vi "标样核查.vi"(11 "标样核查配置":T1={"数据保存间隔"=1.0, "水温标样值"=0.0, "pH标样值"=0.0, "溶解氧标样值"=0.0, "电导率标样值"=0.0, "浊度标样值"=0.0}) -> ()   [LabVIEW 2016, in "国弘多参数.lvlib"]
panel:
  out "运行状态":u16(ring) items=["空闲", "水样测试", "标样核查"]
  out "seconds since 1Jan1904":timestamp
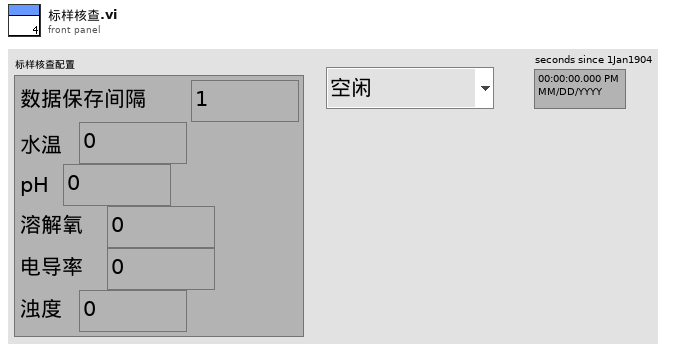
[diagram p1: front panel]
types:
  T1 = cluster{"数据保存间隔":dbl, "水温标样值":dbl, "pH标样值":dbl, "溶解氧标样值":dbl, "电导率标样值":dbl, "浊度标样值":dbl}
  T2 = cluster{"因子编码":string, "单位":string, "标样参考值":sgl, "水样数据时间":timestamp, "水样实测值":sgl, "水样数据标识":string, "探头温度":sgl}
  T3 = typedef "LVDateTimeRec.ctl" = cluster{"秒数的小数部分":dbl, "秒":i32, "分":i32, "时":i32, "日":i32, "月":i32, "年":i32, "天数（周）":i32, "天数（年）":i32, "DST":i32}
  T4 = cluster{"CH":u16, "监测值":dbl, "监测信号值":dbl, "温度偏移修正值":sgl}
  T5 = cluster{"电极状态标志":u16, "电极型号标志":u16, "酸碱度测量值":sgl, "温度测量值":sgl, "酸碱度信号值":sgl, "温度信号值":sgl, "酸碱度偏移修正值":sgl, "温度偏移修正值":sgl, "手动温度补偿值":sgl, "酸碱度电极零点":sgl, "酸碱度电极斜率":sgl, "第1点标准值记录":sgl, "第1点信号值记录":sgl, "第1点温度值记录":sgl, "第2点标准值记录":sgl, "第2点信号值记录":sgl, "第2点温度值记录":sgl, "命令滤波设定":u16, "温度模式":enum16{"ATC", "MTC"}, "生产批次":u16, "电极序号":u16, "串口地址":u16, "串口波特率":enum16{"9600", "19200", "115200"}, "串口校验位":enum16{"NONE", "ODD", "EVEN"}, "串口停止位":enum16{"1bit", "2bit"}, "第一点标准值":sgl, "第二点标准值":sgl}
  T6 = cluster{"电极状态标志":u16, "电极型号标志":u16, "溶解氧测量值":sgl, "温度测量值":sgl, "溶解氧饱和度值":sgl, "盐度补偿值":sgl, "大气压补偿值":sgl, "溶解氧偏移修正值":sgl, "温度偏移修正值":sgl, "手动温度补偿值":sgl, "溶解氧电极零点":sgl, "溶解氧电极斜率":sgl, "第1点标准值记录":sgl, "第1点信号值记录":sgl, "第1点温度值记录":sgl, "第2点标准值记录":sgl, "第2点信号值记录":sgl, "第2点温度值记录":sgl, "命令滤波设定":u16, "温度模式":enum16{"ATC", "MTC"}, "生产批次":u16, "电极序号":u16, "串口地址":u16, "串口波特率":enum16{"9600", "19200", "115200"}, "串口校验位":enum16{"NONE", "ODD", "EVEN"}, "串口停止位":enum16{"1bit", "2bit"}, "第一点标准值":sgl, "第二点标准值":sgl}
  T7 = cluster{"电极状态标志":u16, "电极型号标志":u16, "电导率测量值":sgl, "温度测量值":sgl, "电导率信号值":sgl, "温度信号值":sgl, "温度补偿系数":sgl, "电导率偏移修正值":sgl, "温度偏移修正值":sgl, "手动温度补偿值":sgl, "电导率电极零点":sgl, "电导率电极斜率":sgl, "命令滤波设定":u16, "温度模式":enum16{"ATC", "MTC"}, "生产批次":u16, "电极序号":u16, "串口地址":u16, "串口波特率":enum16{"9600", "19200", "115200"}, "串口校验位":enum16{"NONE", "ODD", "EVEN"}, "串口停止位":enum16{"1bit", "2bit"}, "第一点标准值":sgl, "第二点标准值":sgl}
  T8 = cluster{"电极状态标志":u16, "电极型号标志":u16, "浊度测量值":sgl, "温度测量值":sgl, "浊度信号值":sgl, "浊度偏移修正值":sgl, "温度偏移修正值":sgl, "手动温度补偿值":sgl, "浊度电极零点":sgl, "浊度电极斜率":sgl, "第1点标准值记录":sgl, "第1点信号值记录":sgl, "第1点温度值记录":sgl, "第2点标准值记录":sgl, "第2点信号值记录":sgl, "第2点温度值记录":sgl, "命令滤波设定":u16, "温度模式":enum16{"ATC", "MTC"}, "生产批次":u16, "电极序号":u16, "串口地址":u16, "串口波特率":enum16{"9600", "19200", "115200"}, "串口校验位":enum16{"NONE", "ODD", "EVEN"}, "串口停止位":enum16{"1bit", "2bit"}, "第一点标准值":sgl, "第二点标准值":sgl}
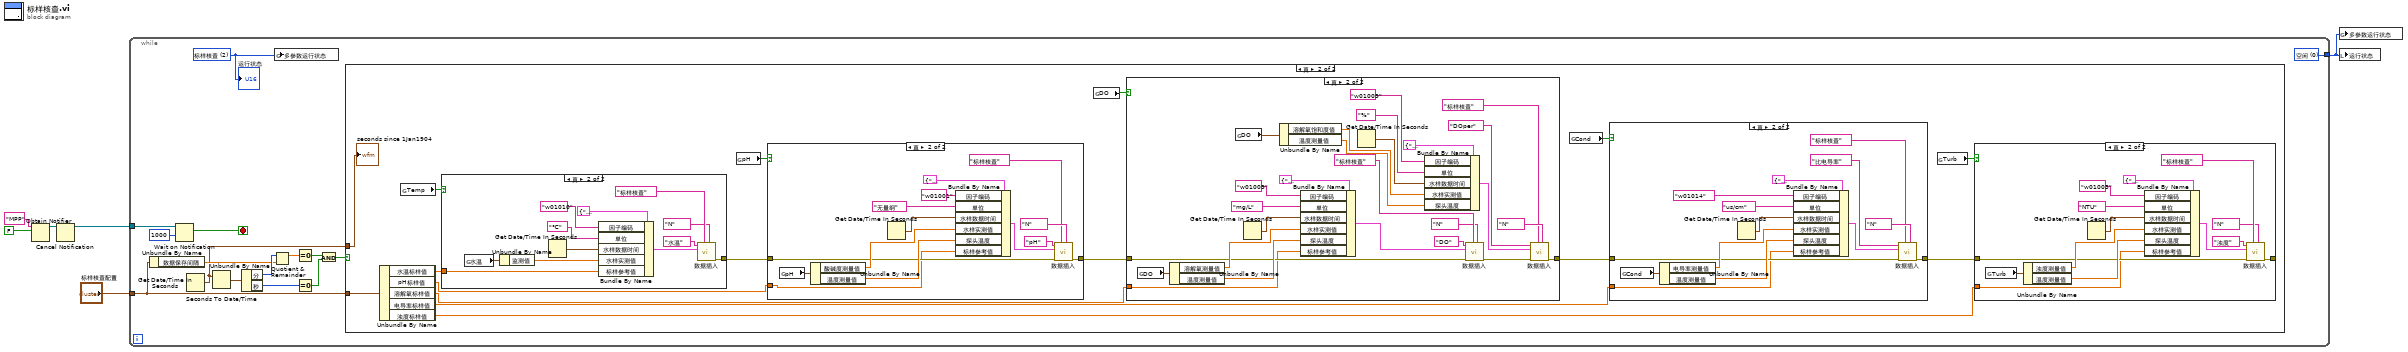
[diagram p0: block diagram]
diagram:
  n1 = Obtain Notifier(name (unnamed)="MPP" ("名称（未命名）"), notification data type=FALSE) -> (notifier out=w2:refnum<notifier>)  [unwired: 2 in, 2 out]
  n2 = Cancel Notification(0:w2) -> (8:w1:refnum<notifier>)  [unwired: 1 in, 2 out]
  n3 = while {
    tunnel: "标样核查配置" -> [w17]
    tunnel: [w11] -> w5
    tunnel: w1 -> [w9]
    stop <- w7 stop-if-true
    w11 = u16 0 items=["空闲", "水样测试", "标样核查"] ("多参数运行状态")
    w10 = u16 2 items=["空闲", "水样测试", "标样核查"] ("多参数运行状态")
    n4 = Unbundle By Name(w17) -> ("数据保存间隔"=w15:dbl)
    n5 = Wait on Notification(notifier=w9, timeout in ms (-1)=1000 ("超时毫秒(-1)")) -> (notification=w7:bool)  [unwired: 2 in, 3 out]
    n6 = Get Date/Time In Seconds() -> (seconds since 1Jan1904=w12:timestamp)
    n7 = Seconds To Date/Time(time stamp (now)=w12) -> (date time rec=w21:T3)  [unwired: 1 in]
    n8 = Unbundle By Name(w21) -> ("分"=w16:i32, "秒"=w20:i32)
    n9 = Quotient & Remainder(x=w16, y=w15) -> (x-y*floor(x/y)=w14:dbl)  [unwired: 1 out]
    n10 = global write "过程全局变量.vi" "多参数运行状态"(w10) -> ()
    n11 = Equal To 0?(x=w14) -> (x = 0?=w13:bool)
    n12 = Equal To 0?(x=w20) -> (x = 0?=w19:bool)
    n13 = And(x=w13, y=w19) -> (x .and. y?=w18:bool)
    n14 = case shown="真" w18 {
      tunnel: w17 -> [_ w27]
      tunnel: w12 -> [_ w37]
      frame False {
      }
      frame True {
        n15 = Unbundle By Name(w27) -> ("水温标样值"=w26:dbl, "pH标样值"=w25:dbl, "溶解氧标样值"=w24:dbl, "电导率标样值"=w23:dbl, "浊度标样值"=w22:dbl)
        n16 = global read "断电保存变量.vi" "Temp"() -> (w32:bool)
        n17 = case shown="真" w32 {
          tunnel: [_ w107] -> w36
          tunnel: w26 -> [_ w106]
          frame False {
          }
          frame True {
            n18 = global read "过程全局变量.vi" "水温"() -> (w116:T4)
            n19 = Unbundle By Name(w116) -> ("监测值"=w115:dbl)
            n20 = Get Date/Time In Seconds() -> (seconds since 1Jan1904=w114:timestamp)
            n21 = Bundle By Name(cluster=T2 {"因子编码"="w01003", "单位"="无量纲", "标样参考值"=0.0, "水样数据时间"=timestamp(0 s since 1904-01-01), "水样实测值"=0.0, "水样数据标识"="N", "探头温度"=0.0} ("data in"), "因子编码"="w01010", "单位"="℃", "水样数据时间"=w114, "水样实测值"=w115, "标样参考值"=w106) -> (w113:T2)
            n22 = call "数据插入.vi"("数据标记表"="N", "测量模式"="标样核查", "data in"=w113, "table输入"="水温") -> ("error out"=w107:errorcluster)  [unwired: 7 in]
          }
        }
        n23 = global read "断电保存变量.vi" "pH"() -> (w31:bool)
        n24 = case shown="真" w31 {
          tunnel: w36 -> [_ w94]
          tunnel: [_ w93] -> w35
          tunnel: w25 -> [_ w92]
          frame False {
          }
          frame True {
            n25 = global read "过程全局变量.vi" "pH"() -> (w100:T5)
            n26 = Unbundle By Name(w100) -> ("酸碱度测量值"=w101:sgl, "温度测量值"=w98:sgl)
            n27 = Get Date/Time In Seconds() -> (seconds since 1Jan1904=w102:timestamp)
            n28 = Bundle By Name(cluster=T2 {"因子编码"="w01003", "单位"="无量纲", "标样参考值"=0.0, "水样数据时间"=timestamp(0 s since 1904-01-01), "水样实测值"=0.0, "水样数据标识"="N", "探头温度"=0.0} ("data in"), "因子编码"="w01001", "单位"="无量纲", "水样数据时间"=w102, "水样实测值"=w101, "探头温度"=w98, "标样参考值"=w92) -> (w103:T2)
            n29 = call "数据插入.vi"("数据标记表"="N", "测量模式"="标样核查", "error in (no error)"=w94, "data in"=w103, "table输入"="pH") -> ("error out"=w93:errorcluster)  [unwired: 6 in]
          }
        }
        n30 = global read "断电保存变量.vi" "DO"() -> (w30:bool)
        n31 = case shown="真" w30 {
          tunnel: w35 -> [_ w80]
          tunnel: [_ w77] -> w34
          tunnel: w24 -> [_ w79]
          frame False {
          }
          frame True {
            n32 = global read "过程全局变量.vi" "DO"() -> (w89:T6)
            n33 = Unbundle By Name(w89) -> ("溶解氧测量值"=w88:sgl, "温度测量值"=w91:sgl)
            n34 = global read "过程全局变量.vi" "DO"() -> (w69:T6)
            n35 = Get Date/Time In Seconds() -> (seconds since 1Jan1904=w87:timestamp)
            n36 = Unbundle By Name(w69) -> ("溶解氧饱和度值"=w70:sgl, "温度测量值"=w67:sgl)
            n37 = Bundle By Name(cluster=T2 {"因子编码"="w01003", "单位"="无量纲", "标样参考值"=0.0, "水样数据时间"=timestamp(0 s since 1904-01-01), "水样实测值"=0.0, "水样数据标识"="N", "探头温度"=0.0} ("data in"), "因子编码"="w01009", "单位"="mg/L", "水样数据时间"=w87, "水样实测值"=w88, "探头温度"=w91, "标样参考值"=w79) -> (w86:T2)
            n38 = Get Date/Time In Seconds() -> (seconds since 1Jan1904=w71:timestamp)
            n39 = Bundle By Name(cluster=T2 {"因子编码"="w01003", "单位"="无量纲", "标样参考值"=0.0, "水样数据时间"=timestamp(0 s since 1904-01-01), "水样实测值"=0.0, "水样数据标识"="N", "探头温度"=0.0} ("data in"), "因子编码"="w01009", "单位"="%", "水样数据时间"=w71, "水样实测值"=w70, "探头温度"=w67) -> (w66:T2)
            n40 = call "数据插入.vi"("数据标记表"="N", "测量模式"="标样核查", "error in (no error)"=w80, "data in"=w86, "table输入"="DO") -> ("error out"=w78:errorcluster)  [unwired: 6 in]
            n41 = call "数据插入.vi"("数据标记表"="N", "测量模式"="标样核查", "error in (no error)"=w78, "data in"=w66, "table输入"="DOper") -> ("error out"=w77:errorcluster)  [unwired: 6 in]
          }
        }
        n42 = global read "断电保存变量.vi" "Cond"() -> (w29:bool)
        n43 = case shown="真" w29 {
          tunnel: w34 -> [_ w54]
          tunnel: [_ w53] -> w33
          tunnel: w23 -> [_ w52]
          frame False {
          }
          frame True {
            n44 = global read "过程全局变量.vi" "Cond"() -> (w60:T7)
            n45 = Unbundle By Name(w60) -> ("电导率测量值"=w61:sgl, "温度测量值"=w58:sgl)
            n46 = Get Date/Time In Seconds() -> (seconds since 1Jan1904=w62:timestamp)
            n47 = Bundle By Name(cluster=T2 {"因子编码"="w01003", "单位"="无量纲", "标样参考值"=0.0, "水样数据时间"=timestamp(0 s since 1904-01-01), "水样实测值"=0.0, "水样数据标识"="N", "探头温度"=0.0} ("data in"), "因子编码"="w01014", "单位"="us/cm", "水样数据时间"=w62, "水样实测值"=w61, "探头温度"=w58, "标样参考值"=w52) -> (w63:T2)
            n48 = call "数据插入.vi"("数据标记表"="N", "测量模式"="标样核查", "error in (no error)"=w54, "data in"=w63, "table输入"="比电导率") -> ("error out"=w53:errorcluster)  [unwired: 6 in]
          }
        }
        n49 = global read "断电保存变量.vi" "Turb"() -> (w28:bool)
        n50 = case shown="真" w28 {
          tunnel: w33 -> [_ w40]
          tunnel: [_ w39] -> _
          tunnel: w22 -> [_ w38]
          frame False {
          }
          frame True {
            n51 = global read "过程全局变量.vi" "Turb"() -> (w49:T8)
            n52 = Unbundle By Name(w49) -> ("浊度测量值"=w48:sgl, "温度测量值"=w51:sgl)
            n53 = Get Date/Time In Seconds() -> (seconds since 1Jan1904=w47:timestamp)
            n54 = Bundle By Name(cluster=T2 {"因子编码"="w01003", "单位"="无量纲", "标样参考值"=0.0, "水样数据时间"=timestamp(0 s since 1904-01-01), "水样实测值"=0.0, "水样数据标识"="N", "探头温度"=0.0} ("data in"), "因子编码"="w01003", "单位"="NTU", "水样数据时间"=w47, "水样实测值"=w48, "探头温度"=w51, "标样参考值"=w38) -> (w46:T2)
            n55 = call "数据插入.vi"("数据标记表"="N", "测量模式"="标样核查", "error in (no error)"=w40, "data in"=w46, "table输入"="浊度") -> ("error out"=w39:errorcluster)  [unwired: 6 in]
          }
        }
        "seconds since 1Jan1904" <- w37
      }
    }
    "运行状态" <- w10
  }
  n56 = global write "过程全局变量.vi" "多参数运行状态"(w5) -> ()
  n57 = local write "运行状态"(w5) -> ()
